vi "clock_nanosleep.vi"(8 "error in (no error)":errorcluster, 9 "flags":T2, 10 "clockid_t":T3=enum."Monotonic", 11 "request":T1) -> (0 "error out":errorcluster, 3 "remain":T1)   [LabVIEW 2013, in "Linux RT Utilities.lvlib"]
uses:
  Linux RT Utilities.lvlib
  Controls/Public/C Structs/timespec_64.ctl
  Controls/Public/C Enums/clockid_t.ctl
  Controls/Public/nanosleep flags.ctl
  Controls/Public/C Structs/timespec_32.ctl
  <vilib>/Utility/error.llb/Error Cluster From Error Code.vi
  <vilib>/NI/NI Linux RT Errno/Public/VIs/Get LV Error Info from Errno.vi
  <vilib>/NI/NI Linux RT Errno/Linux Errno.lvlib
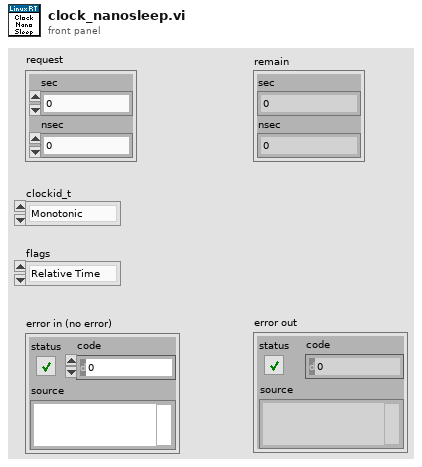
[diagram p1: front panel]
types:
  T1 = typedef "Linux RT Utilities.lvlib/timespec_64.ctl" = cluster{"sec":u64, "nsec":u64}
  T2 = typedef "Linux RT Utilities.lvlib/nanosleep flags.ctl" = enum16{"Relative Time", "Absolute Time"}
  T3 = typedef "Linux RT Utilities.lvlib/clockid_t.ctl" = enum16{"Realtime", "Monotonic"}
  T4 = typedef "Linux RT Utilities.lvlib/timespec_32.ctl" = cluster{"sec":u32, "nsec":u32}
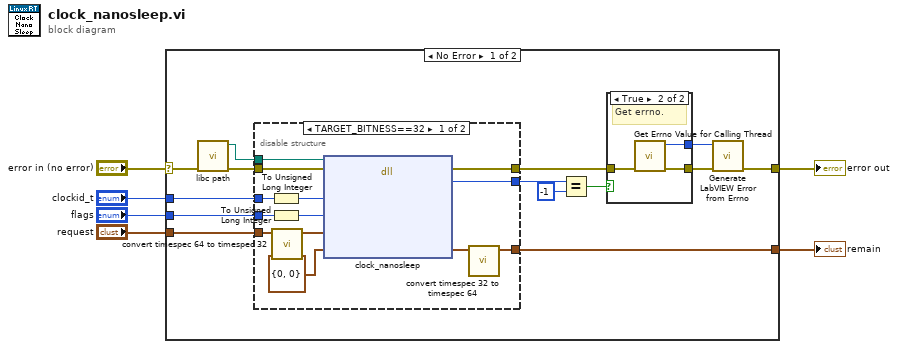
[diagram p0: block diagram]
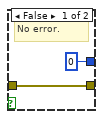
[diagram p2: hidden frame]
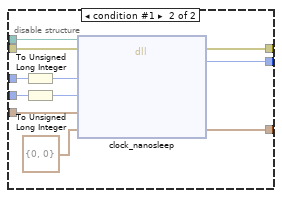
[diagram p3: hidden frame]
diagram:
  n1 = case shown="No Error" "error in (no error)" {
    selector: "error in (no error)" -> [w17 w50]
    tunnel: [w7 w50] -> w5
    tunnel: "request" -> [w18 _]
    tunnel: "clockid_t" -> [w20 _]
    tunnel: "flags" -> [w19 _]
    tunnel: [w14 _] -> w1
    frame No Error {
      n2 = call "libc path.vi"("error in (no error)"=w17) -> ("error out"=w16:errorcluster, "Path"=w15:path)  [unwired: 9 in]
      n3 = disable-structure shown="TARGET_BITNESS==32" {
        disable-tunnel: [w38 w49] -> w9
        disable-tunnel: w20 -> [w37 w48]
        disable-tunnel: w19 -> [w36 w47]
        disable-tunnel: w18 -> [w31 w40]
        disable-tunnel: w16 -> [w30 w43]
        disable-tunnel: w15 -> [w29 w42]
        disable-tunnel: [w27 w41] -> w14
        disable-tunnel: [w26 w39] -> w8
        frame condition #0 (active) {
          n4 = To Unsigned Long Integer(number=w37) -> (unsigned 32bit integer=w35:u32)
          n5 = To Unsigned Long Integer(number=w36) -> (unsigned 32bit integer=w34:u32)
          n6 = call "convert timespec 64 to timespec 32.vi"("timespec 64"=w31) -> ("timespec 32"=w32:T4)  [unwired: 10 in]
          n7 = dll-call lib="?" fn="clock_nanosleep"(path in=w29, error in=w30, "clockid_t"=w35, "flags"=w34, "request"=w32, "remain"=T4 {"sec"=0, "nsec"=0} ("timespec")) -> (error out=w38:errorcluster, "status"=w26:i32, "remain"=w28:T4)  [unwired: 4 in, 1 out]
          n8 = call "convert timespec 32 to timespec 64.vi"("timespec 32"=w28) -> ("timespec 64"=w27:T1)  [unwired: 10 in]
        }
        frame condition #1 {
          n9 = To Unsigned Long Integer(number=w48) -> (unsigned 32bit integer=w46:u32)
          n10 = To Unsigned Long Integer(number=w47) -> (unsigned 32bit integer=w45:u32)
          n11 = dll-call lib="?" fn="clock_nanosleep"(path in=w42, error in=w43, "clockid_t"=w46, "flags"=w45, "request"=w40, "remain"=T1 {"sec"=0, "nsec"=0} ("timespec")) -> (error out=w49:errorcluster, "status"=w39:i32, "remain"=w41:T1)  [unwired: 4 in, 1 out]
        }
      }
      n12 = Equal?(x=w8, y=-1) -> (x = y?=w11:bool)
      n13 = case shown="True" w11 {
        tunnel: w9 -> [w22 w25]
        tunnel: [w22 w24] -> w12
        tunnel: [0 ("errno") w23] -> w13
        frame False {
          # "No error."
        }
        frame True {
          # "Get errno."
          n14 = call <vilib>:"Get Errno Value for Calling Thread.vi"("error in (no error)"=w25) -> ("error out"=w24:errorcluster, "errno"=w23:i32)  [unwired: 9 in]
        }
      }
      n15 = call <vilib>:"Generate LabVIEW Error from Errno.vi"("error in (no error)"=w12, "errno"=w13) -> ("error out"=w7:errorcluster)  [unwired: 9 in]
    }
    frame Error {
    }
  }
  "error out" <- w5
  "remain" <- w1
